vi "AverageIntensity.vi"(8 "error in":errorcluster, 10 "rate (Hz)":dbl=100.0 format="%0.2f", 11 "Time Target (s)":dbl=10.0) -> (0 "error out":errorcluster, 3 "Average intensity (cts/s)":dbl)   [LabVIEW 2011]
uses:
  <vilib>/DAQmx/read.llb/DAQmx Read (Counter 1D U32 1Chan NSamp).vi
  <vilib>/DAQmx/create/channels.llb/DAQmx Create Channel (CI-Count Edges).vi
  <vilib>/DAQmx/configure/timing.llb/DAQmx Timing (Sample Clock).vi
  <vilib>/DAQmx/miscellaneous.llb/DAQmx Fill In Error Info.vi
  Program Files/National Instruments/LabVIEW 2011/resource/objmgr/daqmx.rc
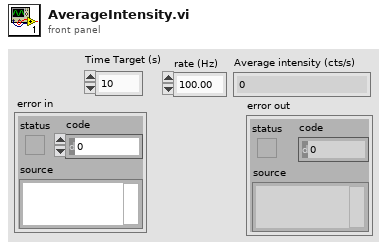
[diagram p1: front panel]
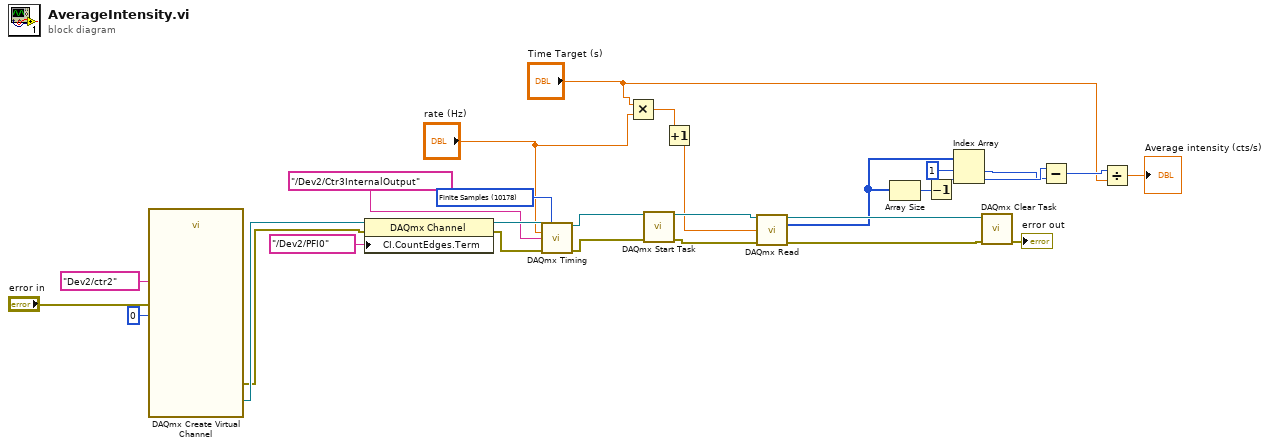
[diagram p0: block diagram]
diagram:
  w20 = 10178 items=["Finite Samples"=10178, "Continuous Samples"=10123, "Hardware Timed Single Point"=12522] ("sample mode")
  n1 = call-poly <vilib>:"DAQmx Create Virtual Channel.vi"("initial count"=u32 0, "counter"=tag "Dev2/ctr2", "error in"="error in") -> ("task out"=w26:refnum<k21>, "error out"=w25:errorcluster)  [unwired: 5 in, 6 out]
  n2 = property class="DAQmx Channel"(reference=w26, error in=w25, "CI.CountEdges.Term"=tag "/Dev2/PFI0") -> (reference out=w24:refnum<k21>, error out=w23:errorcluster)
  n3 = call-poly <vilib>:"DAQmx Timing.vi"("task/channels in"=w24, "sample mode"=w20, "rate"="rate (Hz)", "source"=tag "/Dev2/Ctr3InternalOutput", "error in"=w23) -> ("task out"=w22:refnum<k21>, "error out"=w21:errorcluster)  [unwired: 9 in]
  n4 = Multiply(x="Time Target (s)", y="rate (Hz)") -> (x*y=w14:dbl)
  n5 = call <vilib>:"DAQmx Start Task.vi"("task/channels in"=w22, "error in"=w21) -> ("task out"=w17:refnum<k21>, "error out"=w16:errorcluster)  [unwired: 12 out]
  n6 = Increment(x=w14) -> (x+1=w13:dbl)
  n7 = call-poly <vilib>:"DAQmx Read.vi"("task/channels in"=w17, "number of samples per channel"=w13, "error in"=w16) -> ("task out"=w12:refnum<k21>, "data"=w9:u32[], "error out"=w11:errorcluster)  [unwired: 10 in]
  n8 = Array Size(array=w9) -> (size(s)=w8:i32)
  n9 = Decrement(x=w8) -> (x-1=w7:i32)
  n10 = Index Array(array=w9, index #1=1 ("index"), index #2=w7) -> (element #1=w5:u32, element #2=w6:u32)
  n11 = call <vilib>:"DAQmx Clear Task.vi"("task in"=w12, "error in"=w11) -> ("error out"=→"error out":errorcluster)  [unwired: 13 in]
  n12 = Subtract(x=w6, y=w5) -> (x-y=w4:u32)
  n13 = Divide(x=w4, y="Time Target (s)") -> (x/y=→"Average intensity (cts/s)":dbl)
